vi "Lookup Command Channel.vi"(7 "VolatusAPI in":refnum<class "VolatusAPI.lvclass">, 8 "error in (no error)":errorcluster, 10 "Channel Name":string) -> (0 "error out":errorcluster, 1 "Send Type":T1, 2 "MsgQ":refnum<class "MessageQ.lvclass">, 4 "Owning Task":string, 6 "Owning Node":string)   [LabVIEW 2020, in "VolatusSeq.lvlib"]
uses:
  VolatusSeq.lvlib
  Volatus/VolatusAPI/VolatusAPI.lvclass
  Send Type.ctl
  Volatus/MessageQ/MessageQ.lvclass
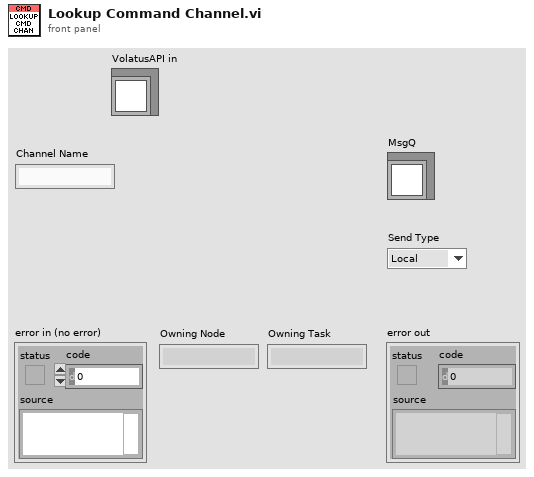
[diagram p1: front panel]
types:
  T1 = typedef "VolatusSeq.lvlib/Send Type.ctl" = enum16{"Local", "Remote"}
  T2 = typedef "VectoConfig.lvlib/Channel Info.ctl" = cluster{"Name":string, "Group":string, "Owning Node":string, "Owning Task":string, "Resource":string}
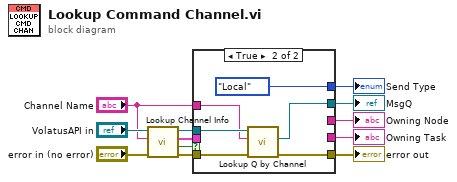
[diagram p0: block diagram]
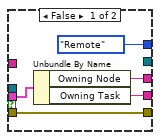
[diagram p2: hidden frame]
diagram:
  n1 = call "Lookup Channel Info.vi"("error in (no error)"="error in (no error)", "Channel Name"="Channel Name", "VolatusAPI in"="VolatusAPI in") -> ("error out"=w10:errorcluster, "Local"=w9:bool, "Channel Info"=w8:T2, "VolatusAPI out"=w7:refnum<class "VolatusAPI.lvclass">)  [unwired: 4 in, 1 out]
  n2 = case shown="True" w9 {
    tunnel: w8 -> [w16 _]
    tunnel: w7 -> [_ w23]
    tunnel: w10 -> [w13 w22]
    tunnel: "Channel Name" -> [_ w21]
    tunnel: [_ w20] -> w5
    tunnel: [Send_Type."Remote" ("Send Type") Send_Type."Local" ("Send Type")] -> w4
    tunnel: [w13 w18] -> w3
    tunnel: [w15 _] -> w2
    tunnel: [w14 _] -> w1
    frame False {
      n3 = Unbundle By Name(w16) -> ("Owning Node"=w15:string, "Owning Task"=w14:string)
    }
    frame True {
      n4 = call "Lookup Q by Channel.vi"("error in (no error)"=w22, "Channel Name"=w21, "VolatusAPI in"=w23) -> ("error out"=w18:errorcluster, "MessageQ"=w20:refnum<class "MessageQ.lvclass">)  [unwired: 5 in, 2 out]
    }
  }
  "error out" <- w3
  "MsgQ" <- w5
  "Send Type" <- w4
  "Owning Node" <- w2
  "Owning Task" <- w1
